vi "RelaySeting.vi"(0 "datain":string[](array[string])=["备注", "负载通道", "负载地址", "延时时间", "output max", "output min", "量测类型", "待测物板号"], 5 "HW CH Number":i32, 7 "Setup":string) -> (4 "REPORT INDECATE":string[][](array[string])=[["微安测试", "", "", "", ""], ["微安量测", "4", "0.000", "0.1", "NG"], ["微安量测", "4", "0.000", "0.1", "NG"], ["微安量测", "4", "0.000", "0.1", "NG"], ["微安量测", "4", "0.000", "0.1", "NG"]], 6 "ROW HEAD":string[](array[string]), 8 "PF":string[](array[string]), 10 "testData":string[](array[string]), 15 "Array":string[](array[string]))   [LabVIEW 2018]
uses:
  Subvi/Global.vi
panel:
  out "数组":bool[](array[boolean])
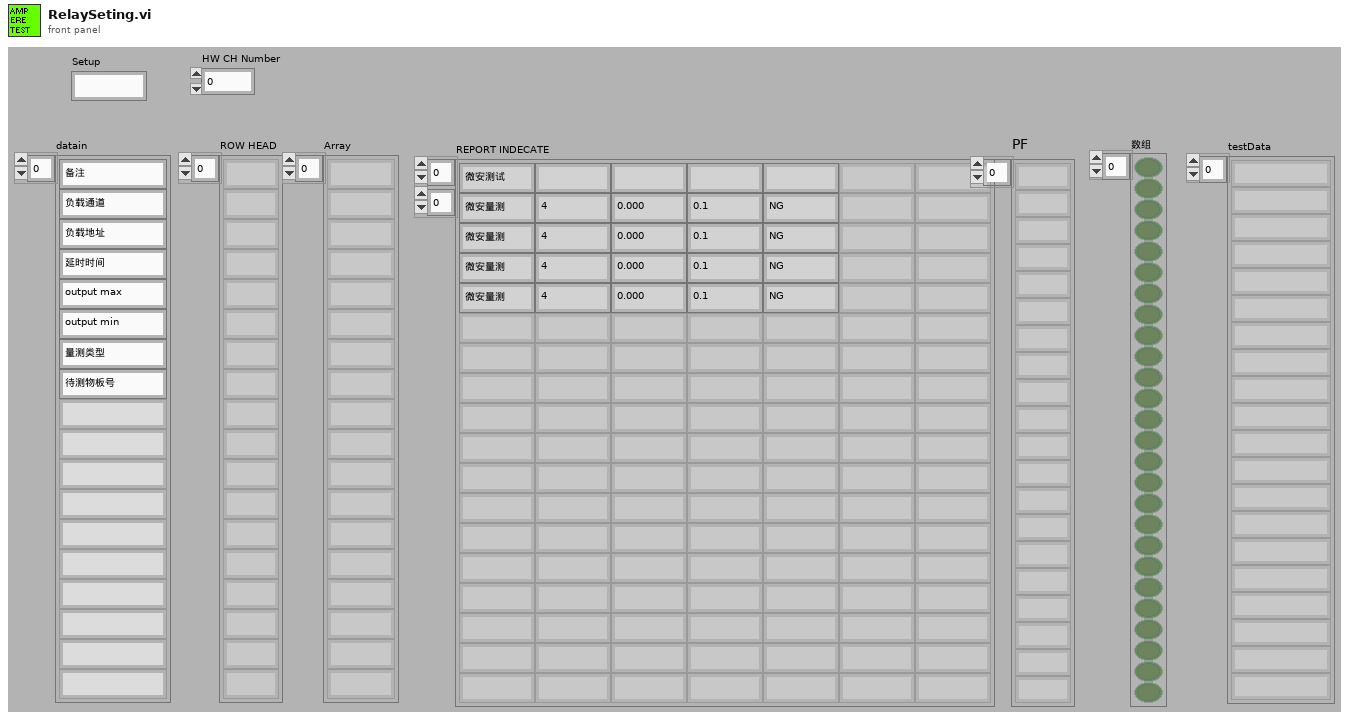
[diagram p1: front panel]
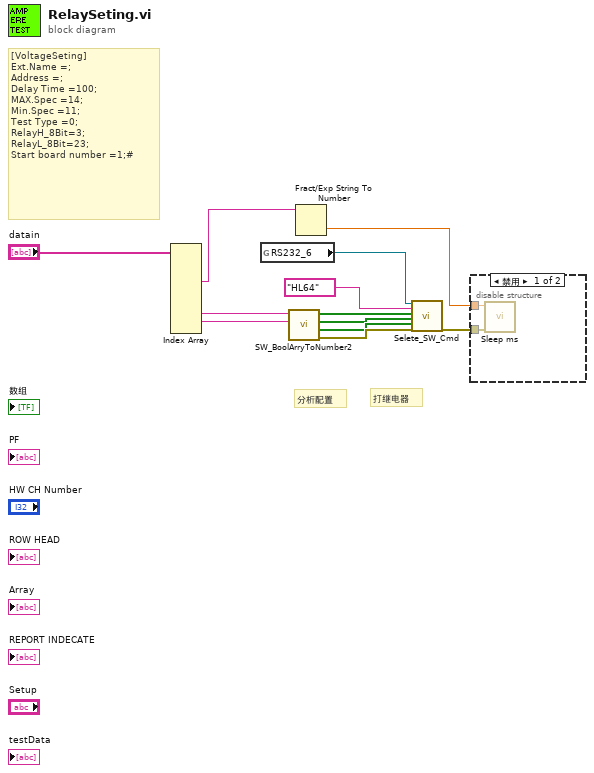
[diagram p0: block diagram]
diagram:
  # "分析配置"
  # "打继电器"
  # "[VoltageSeting]\nExt.Name =;\nAddress =;\nDelay Time =100;\nMAX.Spec =14;\nMin.Spec =11;\nTest Type =0;\nRelayH_8Bit=3;\nRelayL_8Bit=23;\nStart board number =1;#"
  n1 = Index Array(array="datain") -> (element #3=w11:string, element #7=w9:string, element #8=w10:string)  [unwired: 9 in, 6 out]
  n2 = global read "Global.vi" "RS232_6"() -> (w1:refnum<visa-resource-name>)
  n3 = call "SW_BoolArryToNumber2.vi"("L32 INUPT"=w10, "H32 INUPT"=w9) -> ("error out"=w8:errorcluster, "64 SW OUT"=w7:bool[], "L_32"=w6:bool[], "H_32"=w5:bool[])  [unwired: 6 in]
  n4 = Fract/Exp String To Number(string=w11) -> (number=w2:dbl)  [unwired: 3 in, 1 out]
  n5 = call "Selete_SW_Cmd.vi"("VISA资源名称 2"=w1, "组合框"="HL64", "H_32"=w5, "L_32"=w6, "64 SW OUT"=w7, "error in (no error)"=w8) -> ("error out"=w3:errorcluster)  [unwired: 12 in, 1 out]
  n6 = disable-structure shown="禁用" {
    disable-tunnel: w3 -> [w14 _]
    disable-tunnel: w2 -> [w13 _]
    frame Disabled {
      n7 = call "Sleep ms.vi"("error in (no error)"=w14, "等待时间（毫秒）"=w13) -> ()  [unwired: 9 in, 1 out]
    }
    frame Enabled {
    }
  }
